vi "DC Motor.vi"() -> ()   [LabVIEW 2013]
uses:
  Cerebellum/Cerebellum.lvclass
  <vilib>/Utility/file.llb/Application Directory.vi
  <vilib>/Utility/xml.llb/Write to XML File.vi
  <vilib>/Utility/xml.llb/Write to XML File(string).vi
  <vilib>/ptbypt/NI_PtbyPt.lvlib
panel:
  in  "stop":bool
  in  "Active?":bool=TRUE
  out "Motion":cluster{"Vel[n]":dbl, "Ref [n]":dbl}(graph)={"Vel[n]"=4.973797743295939, "Ref [n]"=4.129050746291892}
  out "RSE":dbl[](graph)=[1.6301331934970253, 1.6095102654996758, 1.6093003501296732, 1.6090906025924516, 1.6088810147803332, 1.6086686323929813, 1.6084579474531406, 1.6082474486632148, 1.6080371362181134, 1.607827010311761, 1.6076171210561088, 1.6074062895916978, 1.6071976982535683, 1.6069892767852507, 1.6067810232749309, 1.6065728786426867, 1.6063680026503437, 1.606165104919899, 1.605967202461222, 1.6057734658682838, 1.605523798788761, 1.6052745982980456, 1.6050221410902115, 1.6048294736041093, 1.604580758744075, 1.604335120926036, 1.6040937641195476, 1.6038526651967253, 1.603611197636902, 1.6033677988022796, 1.6031254522107905, 1.6028798552815235, 1.6026936962424172, 1.6024517774742515, 1.6022102937732297, 1.6019691427579164, 1.6017324477639663, 1.6014972635397875, 1.601263404182759, 1.6010336604921718, 1.6008078190640511, 1.6005839860349025, 1.600360340652914, 1.6001368788458898, 1.5999136004090748, 1.59969050513821, 1.5994675928294562, 1.5992448632794494, 1.5990223162852866, 1.5987994975247433, 1.5985748995224027, 1.5983511718479786, 1.5981256005274753, 1.5979006077920408, 1.5976801347832212, 1.5974639441344933, 1.5972480899632286, 1.5970323837985565, 1.59681682343305, 1.5966003788839596, 1.5963811689665808, 1.5961609889525192, 1.5959398943094383, 1.5957181455119773, 1.5954969526424714, 1.5952759377179972, 1.5950552316502238, 1.594836161019277, 1.5946174374547308, 1.5943988601643269, 1.5941804532846635, 1.5939652983535815, 1.5937511125694614, 1.5935409124905462, 1.5933313577665331, 1.593121907623223, 1.5929125606427823, 1.5927033166220594, 1.592494175358014, 1.592283290348263, 1.5920707712983204, 1.5918589636428824, 1.5916472652146405, 1.5914386843533685, 1.5911826955798998, 1.5909281116456757, 1.5906757283716109, 1.590423592063031, 1.590171659133776, 1.5899199286835757, 1.5896650673259456, 1.5894668437142325, 1.5892139806539354, 1.5890193019841228, 1.5887683875753245, 1.5885738685109956, 1.5883202314409217, 1.588120609463274, 1.5879244173338047, 1.5876721101506017, 1.5874727653272962, 1.5872768440407499, 1.5870248612893476, 1.5868257903293845, 1.5866327291538347, 1.5863378133089263, 1.5860951966990438, 1.5858529206517509, 1.585610831053437, 1.5853689262927824, 1.58512720552938, 1.5848856679258678, 1.5846443126479361, 1.5844031388643178, 1.5841621457466837, 1.583921332469766, 1.5836806982112035, 1.583440210249824, 1.583201419592553, 1.5829642176906018, 1.5827271728916188, 1.5824902816397233, 1.5822529211514036, 1.5820139819373482, 1.5817757290769934, 1.5815378624961443, 1.5813027654730716, 1.5810679649240464, 1.5808332972576609, 1.5805992063000687, 1.5803674885822558, 1.5801359260354189, 1.5799069051901904, 1.5796783368708691, 1.579448539910904, 1.579217297799696, 1.578986508506318, 1.5916732108892273, 2.6833301334432385, 2.6806650261161065, 2.6806650261159946, 2.6806650261160003, 2.680665026116, 2.68066502611599, 2.218155515890707, 1.5775806656378726, 1.577406307739928, 1.5772326978769284, 1.5770590405887068, 1.5768853359443393, 1.5767115840115935]
  out "U[n]":T1(graph)={"PD[n]"=0.47343919232495496, "EC[n]"=0.6009713376260425, "PC Right"=0.19077437804195824, -0.05757039754890156, 0.13320398049305668}
  out "3D":refnum<vi>(3d-picture)
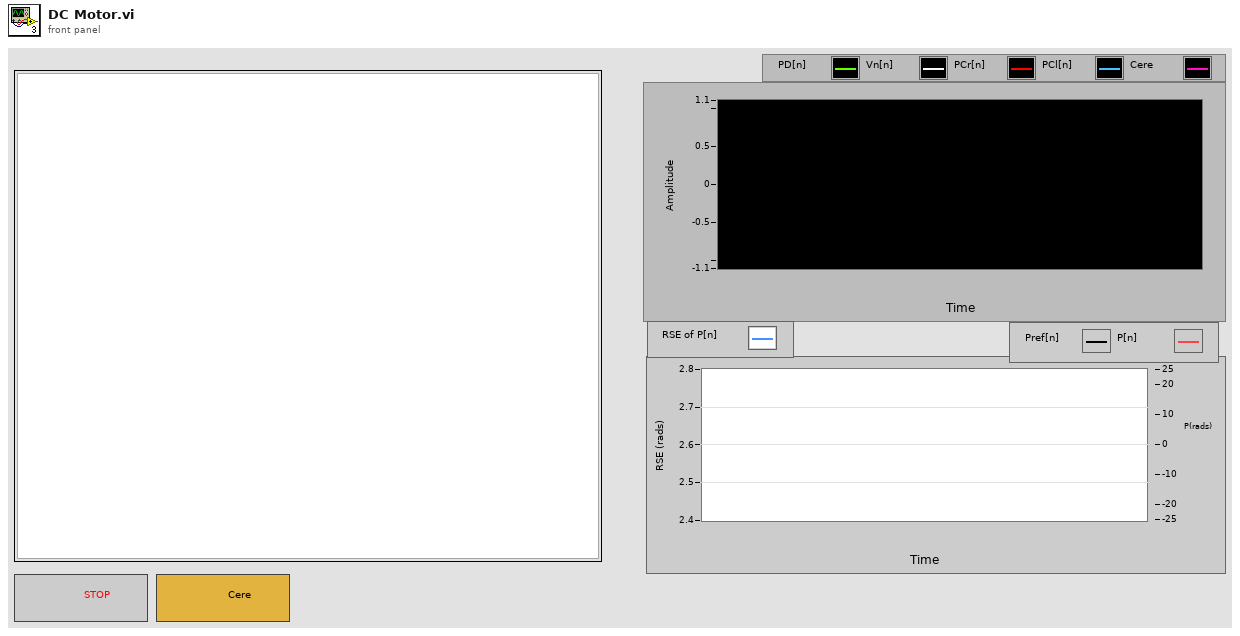
[diagram p1: front panel]
types:
  T1 = cluster{"PD[n]":dbl, "EC[n]":dbl, "PC Right":dbl, dbl, dbl}
  T2 = cluster{"PD[n]":dbl, "EC[n]":dbl, "PC Right":dbl, dbl, dbl}[]
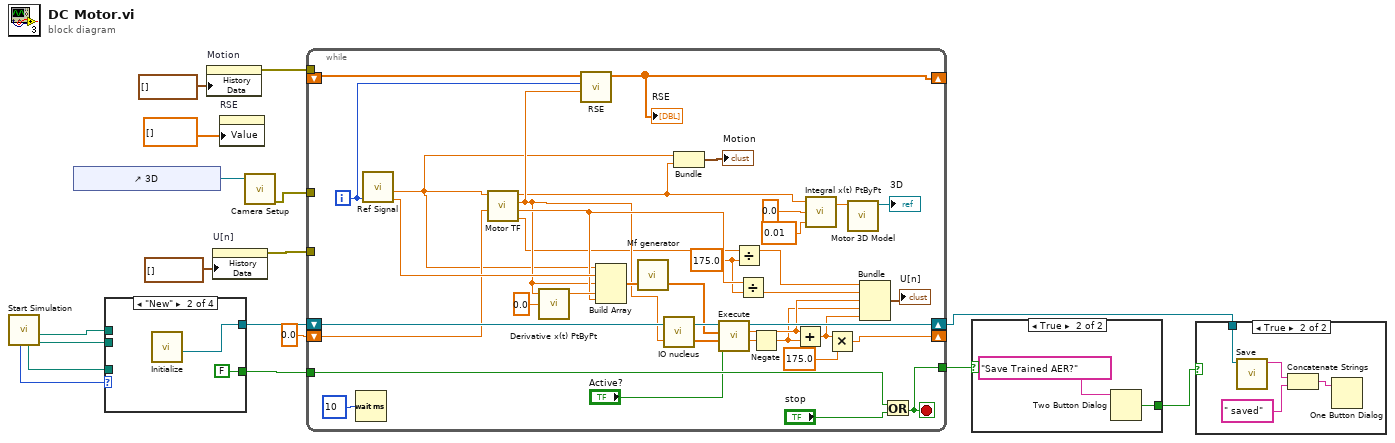
[diagram p0: block diagram]
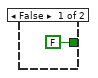
[diagram p3: hidden frame]
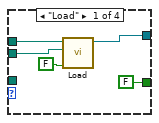
[diagram p4: hidden frame]
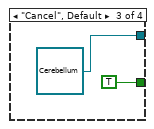
[diagram p5: hidden frame]
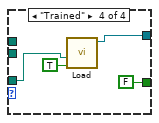
[diagram p6: hidden frame]
diagram:
  n1 = call "Start Simulation.vi"() -> ("Left Hem Path"=w11:path, "Right Hem Path"=w12:path, "TrainedPath"=w2:path, "Action"=w3:enum16{"Trained", "Load", "New", "Cancel"})  [unwired: 8 in]
  n2 = control-ref of="3D"() -> (w17:refnum<vi>)
  n3 = case shown="\"New\"" w3 {
    tunnel: [w22 w24 refnum<class "Cerebellum.lvclass"> refnum ("Cerebellum out") w28] -> w14
    tunnel: w12 -> [w21 _ _ _]
    tunnel: w11 -> [w20 _ _ _]
    tunnel: [FALSE FALSE TRUE FALSE] -> w10
    tunnel: w2 -> [_ _ _ w27]
    frame "Load" {
      n4 = call "Load.vi"("Trained?"=FALSE, "Left Hem Path"=w20, "Right Hem Path"=w21) -> ("Cerebellum out"=w22:refnum<class "Cerebellum.lvclass">)  [unwired: 8 in]
    }
    frame "New" {
      n5 = call "Initialize.vi"() -> ("Cerebellum out"=w24:refnum<class "Cerebellum.lvclass">)  [unwired: 1 in, 3 out]
    }
    frame "Cancel", Default {
    }
    frame "Trained" {
      n6 = call "Load.vi"("Trained?"=TRUE, "Trained Path"=w27) -> ("Cerebellum out"=w28:refnum<class "Cerebellum.lvclass">)  [unwired: 9 in]
    }
  }
  n7 = property on="Motion" class="WFChart (strict)"("History Data"=cluster{"Vel[n]":dbl, "Ref [n]":dbl}[] []) -> (error out=w8:errorcluster)  [unwired: 2 in, 1 out]
  n8 = property on="U[n]" class="WFChart (strict)"("History Data"=T2 []) -> (error out=w15:errorcluster)  [unwired: 2 in, 1 out]
  n9 = property on="RSE" class="WFGraph (strict)"("Value"=dbl[] [] ("Mfs Inputs")) -> ()  [unwired: 2 in, 2 out]
  n10 = call "Camera Setup.vi"("SceneGraphDisplay in"=w17) -> ("error out"=w16:errorcluster)  [unwired: 10 in]
  n11 = while {
    tunnel: w16 -> [_]
    tunnel: w15 -> [_]
    shift-right: [w61] -> w4
    shift-left: w14 -> [w62]
    shift-right: [w47] -> _
    shift-left: 0.0 -> [w54]
    tunnel: w10 -> [w46]
    shift-right: [w41] -> _
    shift-left: _ -> [w42]
    tunnel: w8 -> [_]
    tunnel: [w35] -> w6
    i -> [w44]
    stop <- w35 stop-if-true
    w32 = 175.0 ("y")
    n12 = Wait (ms)(milliseconds to wait=u32 10) -> ()  [unwired: 1 out]
    n13 = call "Ref Signal.vi"("Samples [n]"=w44) -> ("Ref [n]"=w39:dbl, "RefDot [n]"=w57:dbl)  [unwired: 3 in]
    n14 = call "Motor TF.vi"("CereInput"=w54, "Vel ref"=w39) -> ("PD[n]"=w37:dbl, "EC[n]"=w51:dbl, "e[n]"=w43:dbl, "Vel[n]"=w38:dbl)  [unwired: 6 in]
    n15 = call <vilib>:"Derivative x(t) PtByPt.vi"("initial condition"=0.0, "x"=w43) -> ("dx/dt"=w55:dbl)  [unwired: 2 in, 1 out]
    n16 = call "RSE.vi"("e[n]"=w43, "Numeric"=w44, "RSE in"=w42) -> ("RSE out"=w41:dbl[])  [unwired: 8 in]
    "RSE" <- w41
    n17 = Build Array(w39, w57, w43, w55, w51) -> (w53:dbl[])
    n18 = call "Mf generator.vi"("Inputs"=w53) -> ("Mfs Inputs"=w52:dbl[])  [unwired: 2 in]
    n19 = call "IO nucleus.vi"("cf"=w43) -> ("cfs"=w58:dbl[])  [unwired: 2 in]
    n20 = Bundle("Ref [n]"=w39, "Vel[n]"=w38) -> (→"Motion":cluster{"Ref [n]":dbl, "Vel[n]":dbl})  [unwired: 1 in]
    n21 = call "Execute.vi"("Active?"="Active?", "cfs"=w58, "Inputs"=w52, "Cerebellum in"=w62) -> ("PC Left"=w59:dbl, "PC Right"=w49:dbl, "Cerebellum out"=w61:refnum<class "Cerebellum.lvclass">)  [unwired: 5 in]
    n22 = Divide(x=w37, y=w32) -> (x/y=w34:dbl)
    n23 = Divide(x=w51, y=w32) -> (x/y=w33:dbl)
    n24 = Negate(x=w59) -> (-x=w48:dbl)
    n25 = Add(x=w49, y=w48) -> (x+y=w31:dbl)
    n26 = call <vilib>:"Integral x(t) PtByPt.vi"("dt"=0.01, "initial condition"=0.0, "x"=w38) -> ("integral x(t)"=w63:dbl)  [unwired: 1 in, 1 out]
    n27 = Multiply(x=w31, y=175.0) -> (x*y=w47:dbl)
    n28 = call "Motor 3D Model.vi"("Angle (deg)"=w63) -> ("3D Picture Control"=→"3D":refnum<vi>)  [unwired: 10 in]
    n29 = Bundle(w34, w33, "PC Right"=w49, w48, w31) -> (→"U[n]":cluster{dbl, dbl, "PC Right":dbl, dbl, dbl})  [unwired: 1 in]
    n30 = Or(x=w46, y="stop") -> (x .or. y?=w35:bool)
  }
  n31 = case shown="True" w6 {
    tunnel: [FALSE ("T button?") w69] -> w5
    frame False {
    }
    frame True {
      n32 = Two Button Dialog(message="Save Trained AER?") -> (T button?=w69:bool)  [unwired: 2 in]
    }
  }
  n33 = case shown="True" w5 {
    tunnel: w4 -> [_ w74]
    frame False {
    }
    frame True {
      n34 = call "Save.vi"("Cerebellum in"=w74) -> ("File name"=w72:string)  [unwired: 9 in, 1 out]
      n35 = Concatenate Strings(w72, " saved") -> (w73:string)
      n36 = One Button Dialog(message=w73) -> ()  [unwired: 1 in, 1 out]
    }
  }
